vi "Split 1D ARRAY in half.vi"(8 "error in (no error)":errorcluster, 10 "Array in":dbl[](array[numeric])) -> (0 "error out":errorcluster, 1 "Array out (2nd half)":dbl[](array[numeric]), 2 "Array out (1st half)":dbl[](array[numeric]))   [LabVIEW 2019, in "Instrument.DAQ.lvclass"]
uses:
  Instrument.DAQ.lvclass
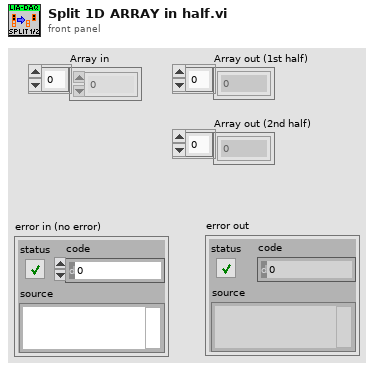
[diagram p1: front panel]
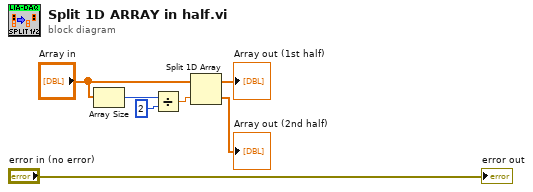
[diagram p0: block diagram]
diagram:
  n1 = Array Size(array="Array in") -> (size(s)=w5:i32)
  n2 = Divide(x=w5, y=2) -> (x/y=w6:dbl)
  n3 = Split 1D Array(array="Array in", index=w6) -> (first subarray=→"Array out (1st half)":dbl[], second subarray=→"Array out (2nd half)":dbl[])
  "error out" <- "error in (no error)"
